vi "ReadBoardInfo.vi"(10 "DeviceInd":u32, 11 "DeviceType":u32) -> (2 "VCI_BOARD_INFO":T1, 3 "success":bool)   [LabVIEW 2011]
uses:
  data/ControlCAN.dll
panel:
  out "VCI_BOARD_INFO_1":T2
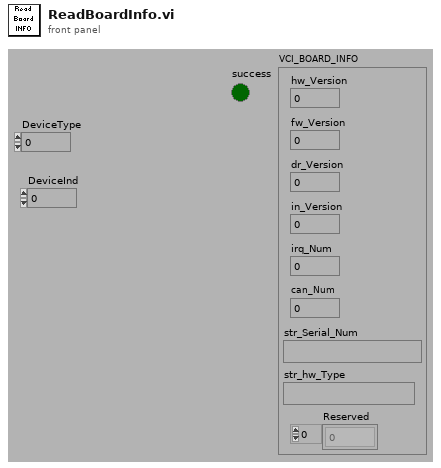
[diagram p1: front panel]
types:
  T1 = cluster{"hw_Version":u16, "fw_Version":u16, "dr_Version":u16, "in_Version":u16, "irq_Num":u16, "can_Num":u8, "str_Serial_Num":string, "str_hw_Type":string, "Reserved":u8[]}
  T2 = cluster{"hw_Version":u16, "fw_Version":u16, "dr_Version":u16, "in_Version":u16, "irq_Num":u16, "can_Num":u8, "str_Serial_Num 0":u8, "str_Serial_Num 1":u8, "str_Serial_Num 2":u8, "str_Serial_Num 3":u8, "str_Serial_Num 4":u8, "str_Serial_Num 5":u8, "str_Serial_Num 6":u8, "str_Serial_Num 7":u8, "str_Serial_Num 8":u8, "str_Serial_Num 9":u8, "str_Serial_Num 10":u8, "str_Serial_Num 11":u8, "str_Serial_Num 12":u8, "str_Serial_Num 13":u8, "str_Serial_Num 14":u8, "str_Serial_Num 15":u8, "str_Serial_Num 16":u8, "str_Serial_Num 17":u8, "str_Serial_Num 18":u8, "str_Serial_Num 19":u8, "str_hw_Type 0":u8, "str_hw_Type 1":u8, "str_hw_Type 2":u8, "str_hw_Type 3":u8, "str_hw_Type 4":u8, "str_hw_Type 5":u8, "str_hw_Type 6":u8, "str_hw_Type 7":u8, "str_hw_Type 8":u8, "str_hw_Type 9":u8, "str_hw_Type 10":u8, "str_hw_Type 11":u8, "str_hw_Type 12":u8, "str_hw_Type 13":u8, "str_hw_Type 14":u8, "str_hw_Type 15":u8, "str_hw_Type 16":u8, "str_hw_Type 17":u8, "str_hw_Type 18":u8, "str_hw_Type 19":u8, "str_hw_Type 20":u8, "str_hw_Type 21":u8, "str_hw_Type 22":u8, "str_hw_Type 24":u8, "str_hw_Type 25":u8, "str_hw_Type 26":u8, "str_hw_Type 27":u8, "str_hw_Type 28":u8, "str_hw_Type 29":u8, "str_hw_Type 30":u8, "str_hw_Type 31":u8, "str_hw_Type 32":u8, "str_hw_Type 33":u8, "str_hw_Type 34":u8, "str_hw_Type 35":u8, "str_hw_Type 36":u8, "str_hw_Type 37":u8, "str_hw_Type 38":u8, "str_hw_Type 39":u8, "Reserved 0":u8, "Reserved 1":u8, "Reserved 2":u8, "Reserved 3":u8}
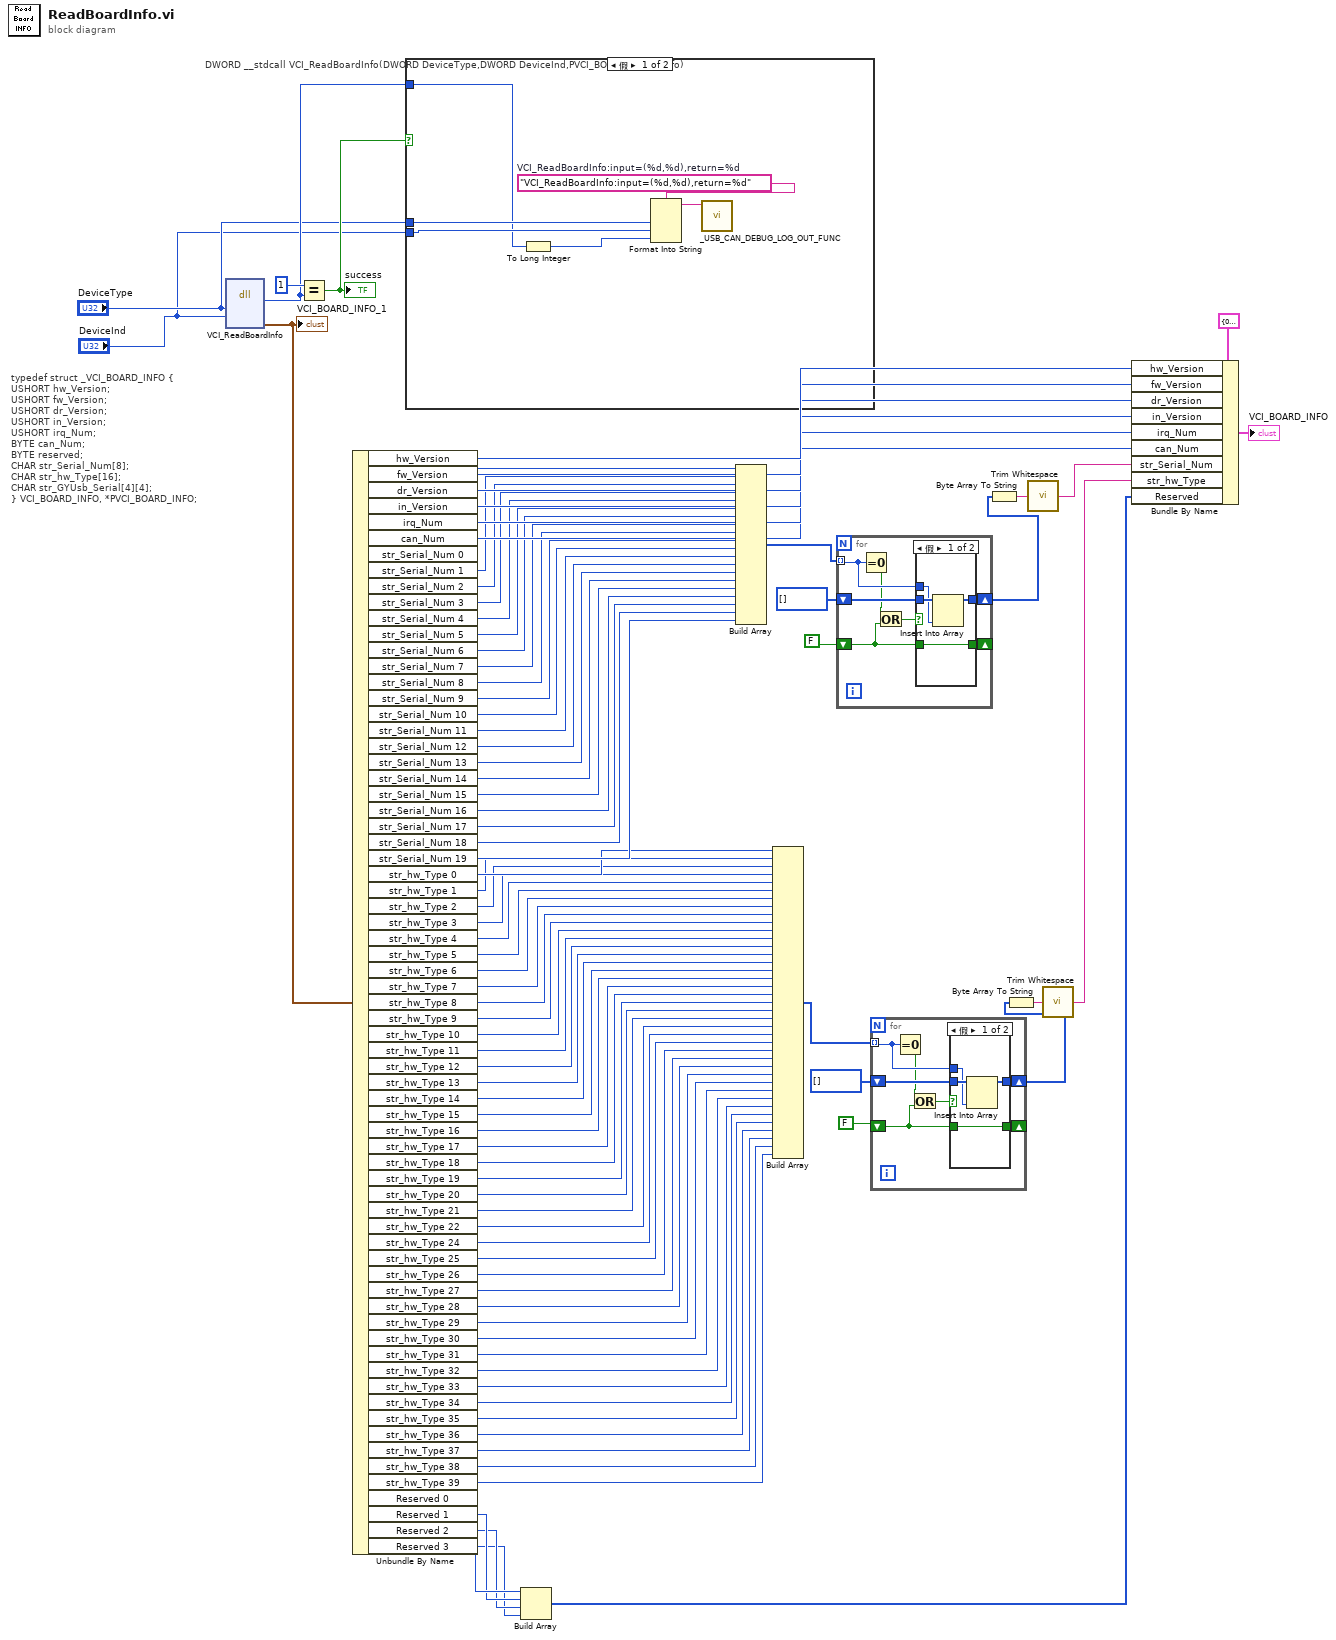
[diagram p0: block diagram]
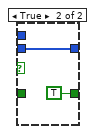
[diagram p3: hidden frame]
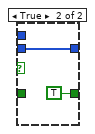
[diagram p4: hidden frame]
diagram:
  # "typedef struct _VCI_BOARD_INFO {\nUSHORT hw_Version;\nUSHORT fw_Version;\nUSHORT dr_Version;\nUSHORT in_Version;\nUSHORT irq_Num;\nBYTE can_Num;\nBYTE reserved;\nCHAR str_Serial_Num[8];\nCHAR str_hw_Type[16];\nCHAR str_GYUsb_Serial[4][4];\n} VCI_BOARD_INFO, *PVCI_BOARD_INFO;"
  # "DWORD __stdcall VCI_ReadBoardInfo(DWORD DeviceType,DWORD DeviceInd,PVCI_BOARD_INFO pInfo)"
  n1 = dll-call lib="PTH1Mabs ZHost_E工作TnewcodeUSB CAN Tool1.97dataControlCAN.dll" fn="VCI_ReadBoardInfo" ("VCI_FindUsbDevice")("DeviceType"="DeviceType", "DeviceInd"="DeviceInd") -> ("返回类型"=w3:u32, "VCI_BOARD_INFO_1"=w14:T2)  [unwired: 6 in, 2 out]
  "VCI_BOARD_INFO_1" <- w14
  n2 = Equal?(x=u32 1, y=w3) -> (x = y?=w4:bool)
  "success" <- w4
  n3 = Unbundle By Name(w14) -> ("hw_Version"=w88:u16, "fw_Version"=w87:u16, "dr_Version"=w86:u16, "in_Version"=w85:u16, "irq_Num"=w84:u16, "can_Num"=w83:u8, "str_Serial_Num 0"=w82:u8, "str_Serial_Num 1"=w81:u8, "str_Serial_Num 2"=w80:u8, "str_Serial_Num 3"=w79:u8, "str_Serial_Num 4"=w78:u8, "str_Serial_Num 5"=w77:u8, "str_Serial_Num 6"=w76:u8, "str_Serial_Num 7"=w75:u8, "str_Serial_Num 8"=w72:u8, "str_Serial_Num 9"=w71:u8, "str_Serial_Num 10"=w70:u8, "str_Serial_Num 11"=w69:u8, "str_Serial_Num 12"=w68:u8, "str_Serial_Num 13"=w67:u8, "str_Serial_Num 14"=w66:u8, "str_Serial_Num 15"=w65:u8, "str_Serial_Num 16"=w64:u8, "str_Serial_Num 17"=w63:u8, "str_Serial_Num 18"=w62:u8, "str_Serial_Num 19"=w61:u8, "str_hw_Type 0"=w59:u8, "str_hw_Type 1"=w58:u8, "str_hw_Type 2"=w57:u8, "str_hw_Type 3"=w56:u8, "str_hw_Type 4"=w55:u8, "str_hw_Type 5"=w54:u8, "str_hw_Type 6"=w53:u8, "str_hw_Type 7"=w52:u8, "str_hw_Type 8"=w51:u8, "str_hw_Type 9"=w50:u8, "str_hw_Type 10"=w49:u8, "str_hw_Type 11"=w48:u8, "str_hw_Type 12"=w47:u8, "str_hw_Type 13"=w46:u8, "str_hw_Type 14"=w45:u8, "str_hw_Type 15"=w44:u8, "str_hw_Type 16"=w43:u8, "str_hw_Type 17"=w42:u8, "str_hw_Type 18"=w41:u8, "str_hw_Type 19"=w40:u8, "str_hw_Type 20"=w39:u8, "str_hw_Type 21"=w38:u8, "str_hw_Type 22"=w37:u8, "str_hw_Type 24"=w36:u8, "str_hw_Type 25"=w35:u8, "str_hw_Type 26"=w34:u8, "str_hw_Type 27"=w33:u8, "str_hw_Type 28"=w32:u8, "str_hw_Type 29"=w31:u8, "str_hw_Type 30"=w30:u8, "str_hw_Type 31"=w29:u8, "str_hw_Type 32"=w28:u8, "str_hw_Type 33"=w27:u8, "str_hw_Type 34"=w26:u8, "str_hw_Type 35"=w25:u8, "str_hw_Type 36"=w24:u8, "str_hw_Type 37"=w23:u8, "str_hw_Type 38"=w22:u8, "str_hw_Type 39"=w21:u8, "Reserved 0"=w20:u8, "Reserved 1"=w19:u8, "Reserved 2"=w18:u8, "Reserved 3"=w17:u8)
  n4 = case shown="假" w4 {
    tunnel: "DeviceType" -> [w95 _]
    tunnel: "DeviceInd" -> [w94 _]
    tunnel: w3 -> [w93 _]
    frame False {
      w91 = "VCI_ReadBoardInfo:input=(%d,%d),return=%d"  # VCI_ReadBoardInfo:input=(%d,%d),return=%d
      n5 = To Long Integer(number=w93) -> (32bit integer=w92:i32)
      n6 = Format Into String(format string=w91, w95, w94, w92) -> (resulting string=w96:string)  [unwired: 2 in, 1 out]
      n7 = call "_USB_CAN_DEBUG_LOG_OUT_FUNC.vi"("Info"=w96) -> ()  [unwired: 11 in]
    }
    frame True {
    }
  }
  n8 = Build Array(w20, w19, w18, w17) -> (w15:u8[])
  n9 = Build Array(w82, w81, w80, w79, w78, w77, w76, w75, w72, w71, w70, w69, w68, w67, w66, w65, w64, w63, w62, w61) -> (w6:u8[])
  n10 = Build Array(w59, w58, w57, w56, w55, w54, w53, w52, w51, w50, w49, w48, w47, w46, w45, w44, w43, w42, w41, w40, w39, w38, w37, w36, w35, w34, w33, w32, w31, w30, w29, w28, w27, w26, w25, w24, w23, w22, w21) -> (w10:u8[])
  n11 = for {
    tunnel: w6 -> [w103] mode=indexing
    shift-right: [w102] -> w5
    shift-left: u8[] [] -> [w101]
    shift-right: [w97] -> _
    shift-left: FALSE -> [w98]
    n12 = Equal To 0?(x=w103) -> (x = 0?=w100:bool)
    n13 = Or(x=w100, y=w98) -> (x .or. y?=w99:bool)
    n14 = case shown="假" w99 {
      tunnel: w103 -> [w106 _]
      tunnel: w101 -> [w107 w109]
      tunnel: [w105 w109] -> w102
      tunnel: w98 -> [w104 _]
      tunnel: [w104 TRUE] -> w97
      frame False {
        n15 = Insert Into Array(array=w107, new element=w106) -> (w105:u8[])  [unwired: 1 in]
      }
      frame True {
      }
    }
  }
  n16 = for {
    tunnel: w10 -> [w116] mode=indexing
    shift-right: [w115] -> w9
    shift-left: u8[] [] -> [w114]
    shift-right: [w110] -> _
    shift-left: FALSE -> [w111]
    n17 = Equal To 0?(x=w116) -> (x = 0?=w113:bool)
    n18 = Or(x=w113, y=w111) -> (x .or. y?=w112:bool)
    n19 = case shown="假" w112 {
      tunnel: w116 -> [w119 _]
      tunnel: w114 -> [w120 w122]
      tunnel: [w118 w122] -> w115
      tunnel: w111 -> [w117 _]
      tunnel: [w117 TRUE] -> w110
      frame False {
        n20 = Insert Into Array(array=w120, new element=w119) -> (w118:u8[])  [unwired: 1 in]
      }
      frame True {
      }
    }
  }
  n21 = Byte Array To String(unsigned byte array=w5) -> (string=w74:string)
  n22 = Byte Array To String(unsigned byte array=w9) -> (string=w60:string)
  n23 = call <vilib>:"Trim Whitespace.vi"("string"=w74) -> ("trimmed string"=w73:string)  [unwired: 1 in]
  n24 = call <vilib>:"Trim Whitespace.vi"("string"=w60) -> ("trimmed string"=w16:string)  [unwired: 1 in]
  n25 = Bundle By Name(cluster=T1 {"hw_Version"=0, "fw_Version"=0, "dr_Version"=0, "in_Version"=0, "irq_Num"=0, "can_Num"=0, "str_Serial_Num"="", "str_hw_Type"="", "Reserved"=[]} ("VCI_BOARD_INFO"), "hw_Version"=w88, "fw_Version"=w87, "dr_Version"=w86, "in_Version"=w85, "irq_Num"=w84, "can_Num"=w83, "str_Serial_Num"=w73, "str_hw_Type"=w16, "Reserved"=w15) -> (→"VCI_BOARD_INFO":T1)
